vi "OperateDatabase.vi"(8 "error in (no error)":errorcluster, 10 "Person in":refnum<class "Person.lvclass">, 11 "State_User in":refnum<class "State_User.lvclass">) -> (0 "error out":errorcluster, 2 "Person out":refnum<class "Person.lvclass">, 3 "State_User out":refnum<class "State_User.lvclass">)   [LabVIEW 2014, in "State_User.lvclass"]
uses:
  State_User.lvclass
  Person_Class/Person.lvclass
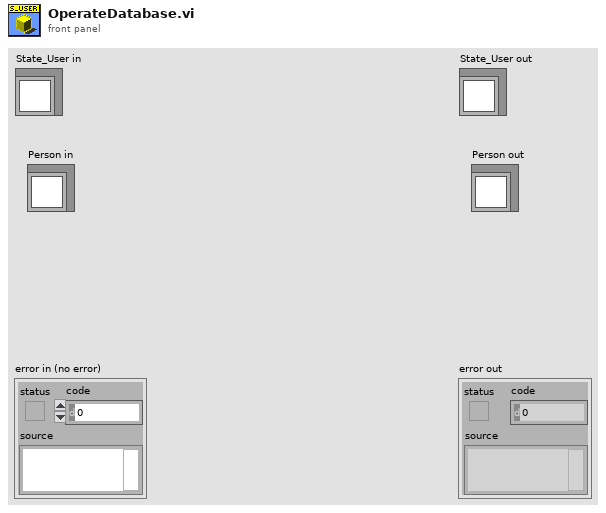
[diagram p1: front panel]
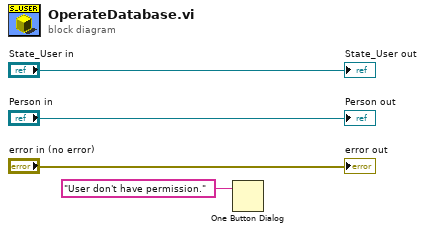
[diagram p0: block diagram]
diagram:
  n1 = One Button Dialog(message="User don't have permission.") -> ()  [unwired: 1 in, 1 out]
  "error out" <- "error in (no error)"
  "State_User out" <- "State_User in"
  "Person out" <- "Person in"
